vi "Async Loop.vi"(8 "error in (no error)":errorcluster, 10 "Process Data":T1, 11 "Path":path) -> (0 "error out":errorcluster)   [LabVIEW 2017, in "Shared Variables CD 2.0 Engine.lvlib"]
uses:
  Shared Variables CD 2.0 Engine.lvlib
  <vilib>/NI Veristand/Custom Device Tools/Custom Device Utility Library/Custom Device Utility Library.lvlib
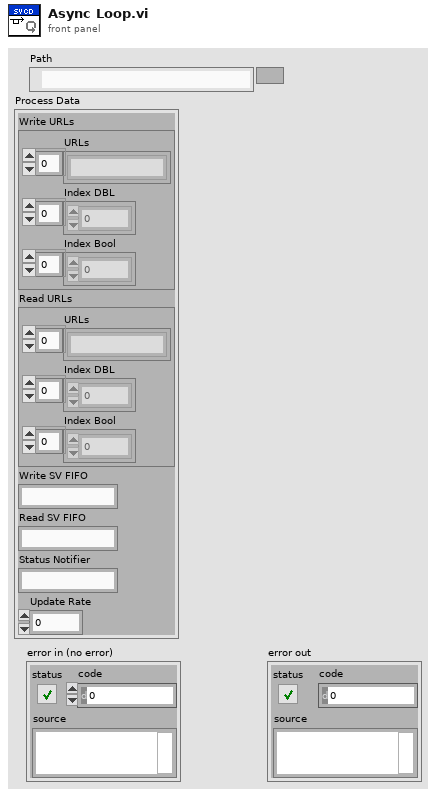
[diagram p1: front panel]
types:
  T1 = cluster{"Write URLs":cluster{"URLs":string[], "Index DBL":i32[], "Index Bool":i32[]}, "Read URLs":cluster{"URLs":string[], "Index DBL":i32[], "Index Bool":i32[]}, "Write SV FIFO":string, "Read SV FIFO":string, "Status Notifier":string, "Update Rate":u32}
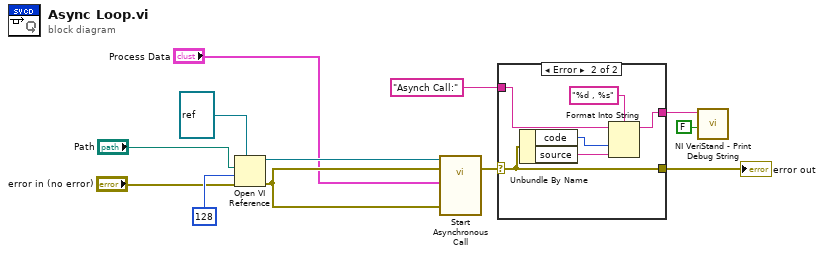
[diagram p0: block diagram]
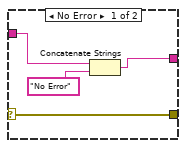
[diagram p2: hidden frame]
diagram:
  n1 = Open VI Reference(type specifier VI Refnum (for type only)=refnum<vi> refnum, vi path="Path", options=128, error in (no error)="error in (no error)") -> (vi reference=w11:refnum<vi>, error out=w10:errorcluster)  [unwired: 2 in]
  n2 = call-by-ref "Start Asynchronous Call"(reference=w11, error in=w10, 8:"error in (no error)"=w10, "Process Data"="Process Data") -> (error out=w6:errorcluster)  [unwired: 9 in, 2 out]
  n3 = case shown="Error" w6 {
    selector: w6 -> [w16 w21]
    tunnel: [w16 w21] -> w5
    tunnel: "Asynch Call:" ("Message") -> [w15 w22]
    tunnel: [w13 w17] -> w3
    frame No Error {
      n4 = Concatenate Strings(w15, "No Error" ("string")) -> (w13:string)
    }
    frame Error {
      n5 = Unbundle By Name(w21) -> ("code"=w20:i32, "source"=w19:string)
      n6 = Format Into String(format string="%d , %s", initial string=w22, w20, w19) -> (resulting string=w17:string)  [unwired: 1 in, 1 out]
    }
  }
  "error out" <- w5
  n7 = call <vilib>:"NI VeriStand - Print Debug String.vi"("Add to log file? (T)"=FALSE, "Message"=w3) -> ()  [unwired: 9 in, 1 out]
